vi "Create.vi"(8 "Error In":errorcluster, 11 "reference in":refnum<class "DBC Communicator.lvclass">) -> (0 "Error Out":errorcluster, 3 "reference out":refnum<class "DBC Communicator.lvclass">)   [LabVIEW 2025, in "DBC Communicator.lvclass"]
uses:
  DBC Communicator.lvclass
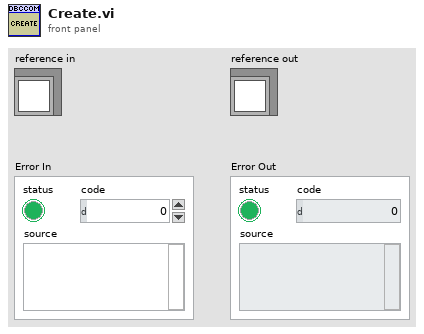
[diagram p1: front panel]
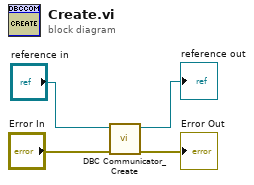
[diagram p0: block diagram]
diagram:
  n1 = call "DBC Communicator_Create.vi"("Error In"="Error In", "reference in"="reference in") -> ("Error Out"=→"Error Out":errorcluster, "reference out"=→"reference out":refnum<class "DBC Communicator.lvclass">)  [unwired: 8 in]
